vi "SendTcpMaskCommand.vi"(6 "機器番号":u8, 9 "InOut?":string(combo), 10 "Sample Name":string="Sample", 11 "アドレス":string) -> (1 "送信文字列":string, 2 "空?":bool, 3 "Send List Out":cluster{"Address":string, "Data":string}[](array[cluster]))   [LabVIEW 2021]
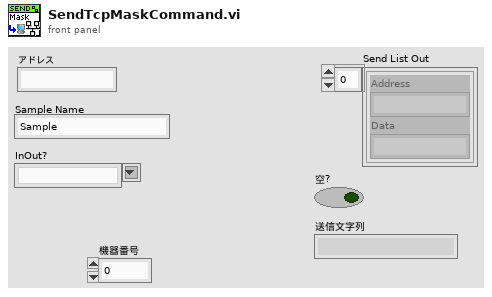
[diagram p1: front panel]
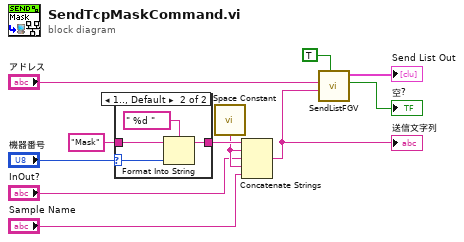
[diagram p0: block diagram]
diagram:
  n1 = case shown="1.., Default" "機器番号" {
    selector: "機器番号" -> [_ w14]
    tunnel: [w12 w16] -> w5
    tunnel: "Mask" ("要素") -> [w12 w13]
    frame 0 {
    }
    frame 1.., Default {
      n2 = Format Into String(format string=" %d " ("形式文字列"), initial string=w13, w14) -> (resulting string=w16:string)  [unwired: 1 in, 1 out]
    }
  }
  n3 = call <vilib>:"Space Constant.vi"() -> ("String"=w2:string)
  n4 = Concatenate Strings(w5, w2, "InOut?", w2, "Sample Name") -> (w4:string)
  "送信文字列" <- w4
  n5 = call "SendListFGV.vi"("Set"=TRUE, "Data"=w4, "アドレス"="アドレス") -> ("空?"=→"空?":bool, "Send List Out"=→"Send List Out":cluster{"Address":string, "Data":string}[])  [unwired: 6 in, 1 out]
